vi "Motor Controller Drive Command.vi"(0 "COM port":refnum<visa-resource-name>, 5 "RS-485 addr.":u8, 7 "Command":string(combo)="R", 9 "RPM setpoint":sgl, 11 "Close port after action":bool) -> (4 "COM port out":refnum<visa-resource-name>, 15 "Error out":errorcluster)   [LabVIEW 2020]
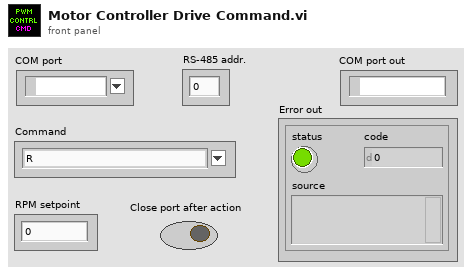
[diagram p1: front panel]
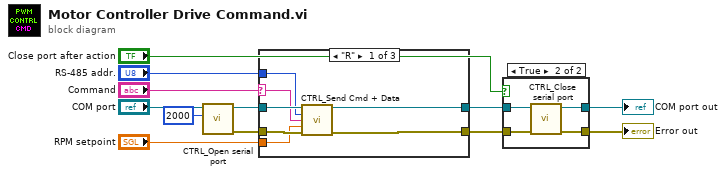
[diagram p0: block diagram]
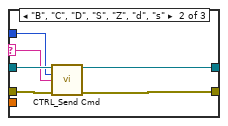
[diagram p3: hidden frame]
diagram:
  n1 = call "CTRL_Open serial port.vi"("timeout (ms)"=u32 2000, "VISA resource name"="COM port") -> ("Error out"=w9:errorcluster, "VISA resource name out"=w10:refnum<visa-resource-name>)  [unwired: 8 in]
  n2 = case shown="\"R\"" "Command" {
    selector: "Command" -> [w16 w23 _]
    tunnel: w10 -> [w19 w25 w27]
    tunnel: w9 -> [w18 w24 w26]
    tunnel: "RPM setpoint" -> [w17 _ _]
    tunnel: [w15 w22 w27] -> w5
    tunnel: [w14 w21 w26] -> w6
    tunnel: "RS-485 addr." -> [w13 w20 _]
    frame "R" {
      n3 = call "CTRL_Send Cmd + Data.vi"("Port"=w19, "RS-485 addr."=w13, "Cmd"=w16, "Data"=w17, "Error In"=w18) -> ("Port out"=w15:refnum<visa-resource-name>, "Error Out"=w14:errorcluster)  [unwired: 9 in]
    }
    frame "B", "C", "D", "S", "Z", "d", "s" {
      n4 = call "CTRL_Send Cmd.vi"("Port"=w25, "RS-485 addr."=w20, "Cmd"=w23, "Error In"=w24) -> ("Port out"=w22:refnum<visa-resource-name>, "Error Out"=w21:errorcluster)  [unwired: 10 in]
    }
    frame Default {
    }
  }
  n5 = case shown="True" "Close port after action" {
    tunnel: [w29 w32] -> w4
    tunnel: w5 -> [w28 w30]
    tunnel: w6 -> [w29 w31]
    tunnel: [w28 w30] -> w1
    frame False {
    }
    frame True {
      n6 = call "CTRL_Close serial port.vi"("Error in"=w31, "VISA resource name"=w30) -> ("Error out"=w32:errorcluster)  [unwired: 9 in]
    }
  }
  "Error out" <- w4
  "COM port out" <- w1
